vi "Slow Rate.vi"(8 "error in (no error)":errorcluster, 11 "ScrollingList in":refnum<class "ScrollingList.lvclass">) -> (0 "error out":errorcluster, 3 "ScrollingList out":refnum<class "ScrollingList.lvclass">)   [LabVIEW 2020, in "ScrollingList.lvclass"]
uses:
  ScrollingList.lvclass
  ScrollingList.lvclass/ScrollingList.ctl
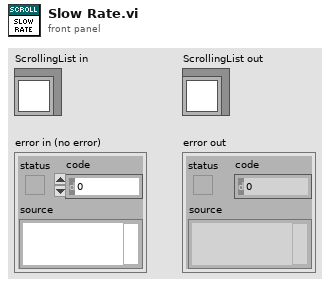
[diagram p1: front panel]
types:
  T1 = typedef "ScrollingList.lvclass/State Data.ctl" = cluster{"Timeout":i32, "Time":timestamp, "Y":i32, "Origin:Top":i16, "Rate":dbl, "ListItems":string[], "Item Height":i32, "Max Height":i32}
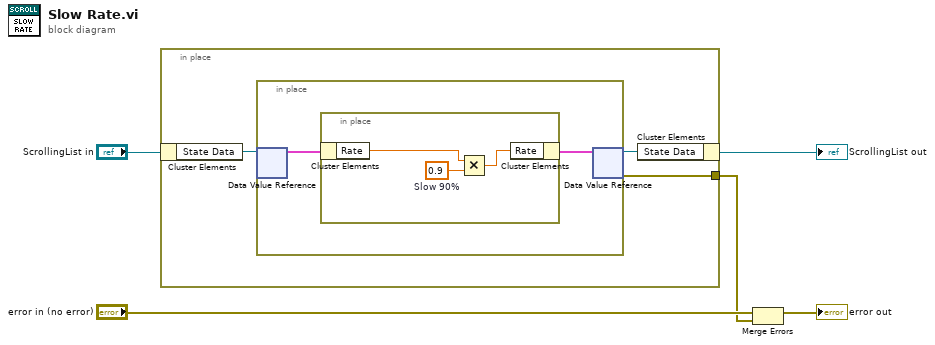
[diagram p0: block diagram]
diagram:
  n1 = in-place {
    in-place-border: [w6] -> w1
    n2 = in-place-cluster #1("ScrollingList in") -> ("State Data"=w8:refnum<data-value>)
    n3 = in-place {
      n4 = in-place-dvr #2(w8) -> (w10:T1)  [unwired: 1 out]
      n5 = in-place {
        w13 = 0.9  # Slow 90%
        n6 = in-place-cluster #3(w10) -> ("Rate"=w12:dbl)
        n7 = Multiply(x=w12, y=w13) -> (x*y=w11:dbl)
        n8 = in-place-cluster #3("Rate"=w11) -> (w9:T1)
      }
      n9 = in-place-dvr #2(w9) -> (w7:refnum<data-value>, w6:errorcluster)
    }
    n10 = in-place-cluster #1("State Data"=w7) -> (→"ScrollingList out":refnum<class "ScrollingList.lvclass">)
  }
  n11 = Merge Errors("error in (no error)", w1) -> (→"error out":errorcluster)
